vi "Extract Index from Ctrl Label.vi"(8 "error in (no error)":errorcluster, 10 "Prefix":string, 11 "Ctl Refnum":refnum<vi>) -> (0 "error out":errorcluster, 3 "Numeric":i32)   [LabVIEW 2016, in "Common.lvlib"]
uses:
  <userlib>/Common Components/Common/Common.lvlib
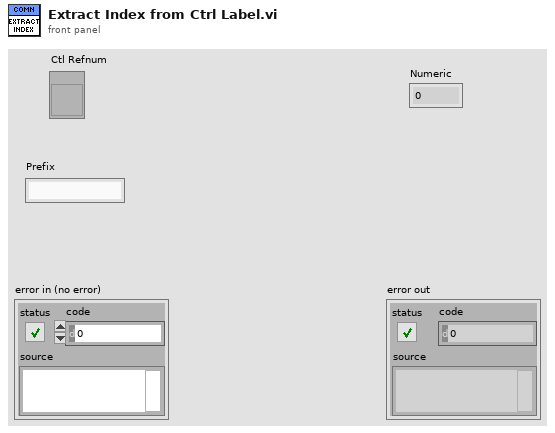
[diagram p1: front panel]
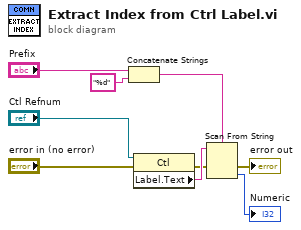
[diagram p0: block diagram]
diagram:
  n1 = Concatenate Strings("Prefix", "%d" ("string")) -> (w4:string)
  n2 = property class="Ctl"(reference="Ctl Refnum", error in="error in (no error)") -> (error out=w1:errorcluster, "Label.Text"=w8:string)  [unwired: 1 out]
  n3 = Scan From String(format string=w4, input string=w8, error in=w1) -> (error out=→"error out":errorcluster, output 1=→"Numeric":i32)  [unwired: 2 in, 2 out]
